vi "BRig_FPGA_v3,95__PortC.vi"() -> ()   [LabVIEW 2014]
uses:
  <vilib>/rvi/Emulation/niFpgaGetClockAttributes.vi
  <vilib>/rvi/Emulation/niFpgaSctlEmulationGetInTimedLoop.vi
  <vilib>/rvi/Emulation/niFpgaEmulationReportErrorSimple.vi
  <vilib>/rvi/eio/common/nirviEmuTemplateMethod_errors.vi
  <vilib>/rvi/Emulation/niFpgaCriticalErrorInLSC.vi
  <vilib>/eio/EIONode/EIONode.xnode
panel:
  out "AnaIn_1_0":i16
  out "AnaIn_1_1":i16
  out "AnaIn_1_2":i16
  out "AnaIn_1_3":i16
  out "AnaIn_1_4":i16
  out "AnaIn_0_4":i16
  out "AnaIn_0_3":i16
  out "AnaIn_0_2":i16
  out "AnaIn_0_1":i16
  out "AnaIn_0_0":i16
  in  "AI_newCycleFlag":bool
  in  "AnaOut1_Pair":u16
  in  "AnaOut0_Pair":u16
  out "fpga_solenoid_R":bool
  out "fpga_solenoid_L":bool
  out "fpga_laser2":bool
  out "fpga_laser1":bool
  in  "L2Led_ON":bool
  in  "L1Led_ON":bool
  in  "Rising(F)_or_Falling(T)":bool
  in  "Solenoid_trig_R":bool
  in  "Solenoid_trig_L":bool
  in  "Solenoid_nTotal_R":u32=100
  in  "Solenoid_nTotal_L":u32=100
  in  "L2Led_Baseline":bool
  in  "L1Led_Baseline":bool
  in  "CueLed_Baseline":bool
  in  "I_allReward":bool
  in  "AnaOut_1":i16
  in  "CueLed_Event":bool
  in  "CueLed_nValley":u32=100
  in  "CueLed_nPeak":u32=100
  in  "LC_Event_l2":bool
  in  "LC_Laser_l2":bool
  in  "LC_nShutter_l2":u32=100
  in  "LC_nValley_l2":u32=100
  in  "LC_nPeak_l2":u32=100
  in  "LR_wrong_nDelay_l2":u32
  in  "LR_reward_nDelay_l2":u32
  in  "LR_wrong_nTotal_l2":u32=100
  in  "LR_reward_nTotal_l2":u32=100
  in  "LR_wrong_laser_l2":bool
  in  "LR_wrong_Event_l2":bool
  in  "LR_reward_Laser_l2":bool
  in  "LR_reward_Event_l2":bool
  out "timeTrial_count":u32
  in  "timeTrial_trig":bool
  in  "k1__counter_per_ms":u16=100 min=100 max=40000 step=1
  in  "LC_nShutter_l1":u32=100
  in  "AnaOut_0":i16
  in  "LC_nValley_l1":u32=100
  in  "LC_nPeak_l1":u32=100
  in  "LC_Event_l1":bool
  in  "LR_wrong_nTotal_l1":u32=100
  in  "LR_wrong_nDelay_l1":u32
  in  "LR_reward_nTotal_l1":u32=100
  in  "LR_reward_nDelay_l1":u32
  in  "LR_reward_Event_l1":bool
  in  "LR_wrong_Event_l1":bool
  out "SelectWrong":bool
  out "SelectReward":bool
  in  "LR_wrong_Laser_l1":bool
  in  "LR_reward_Laser_l1":bool
  in  "Left(F)_or_Right(T)":bool
  in  "ignoreWrong":bool
  in  "SelectionState":bool
  in  "LC_Laser_l1":bool
  in  "FPGA_Stop":bool
  in  "audioTrigger_L":bool
  in  "audioTrigger_R":bool
  in  "audioFreq_L_kHz":u8=14 min=1 max=14 step=1
  in  "audioAmp_L":u16=1 min=1 max=32767 step=1
  in  "audioFreq_R_kHz":u8=14 min=1 max=14 step=1
  in  "audioAmp_R":u16=1 min=1 max=32767 step=1
  in  "A3_SL":bool
  in  "A1_SR":bool
  in  "Counts_Reset":bool
  out "A4_LickR":u32
  out "A2_LickL":u32
  in  "A6_Act":bool
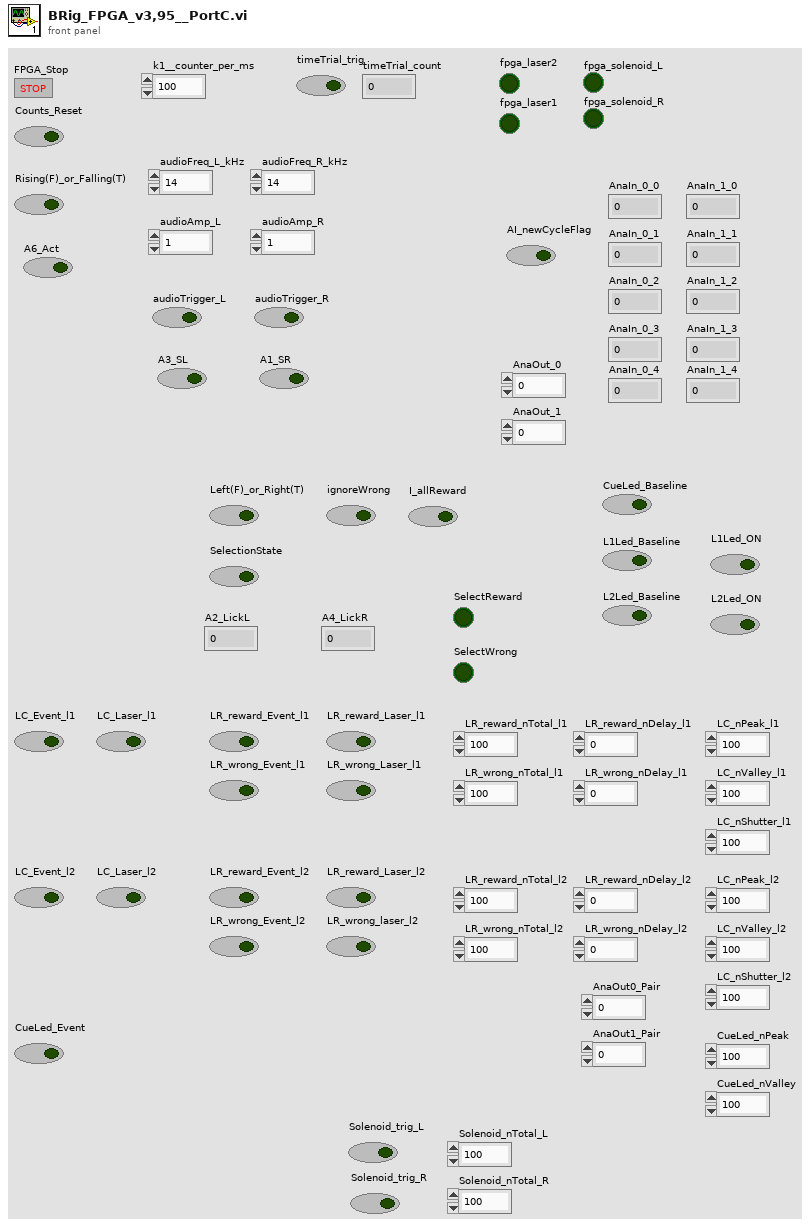
[diagram p1: front panel]
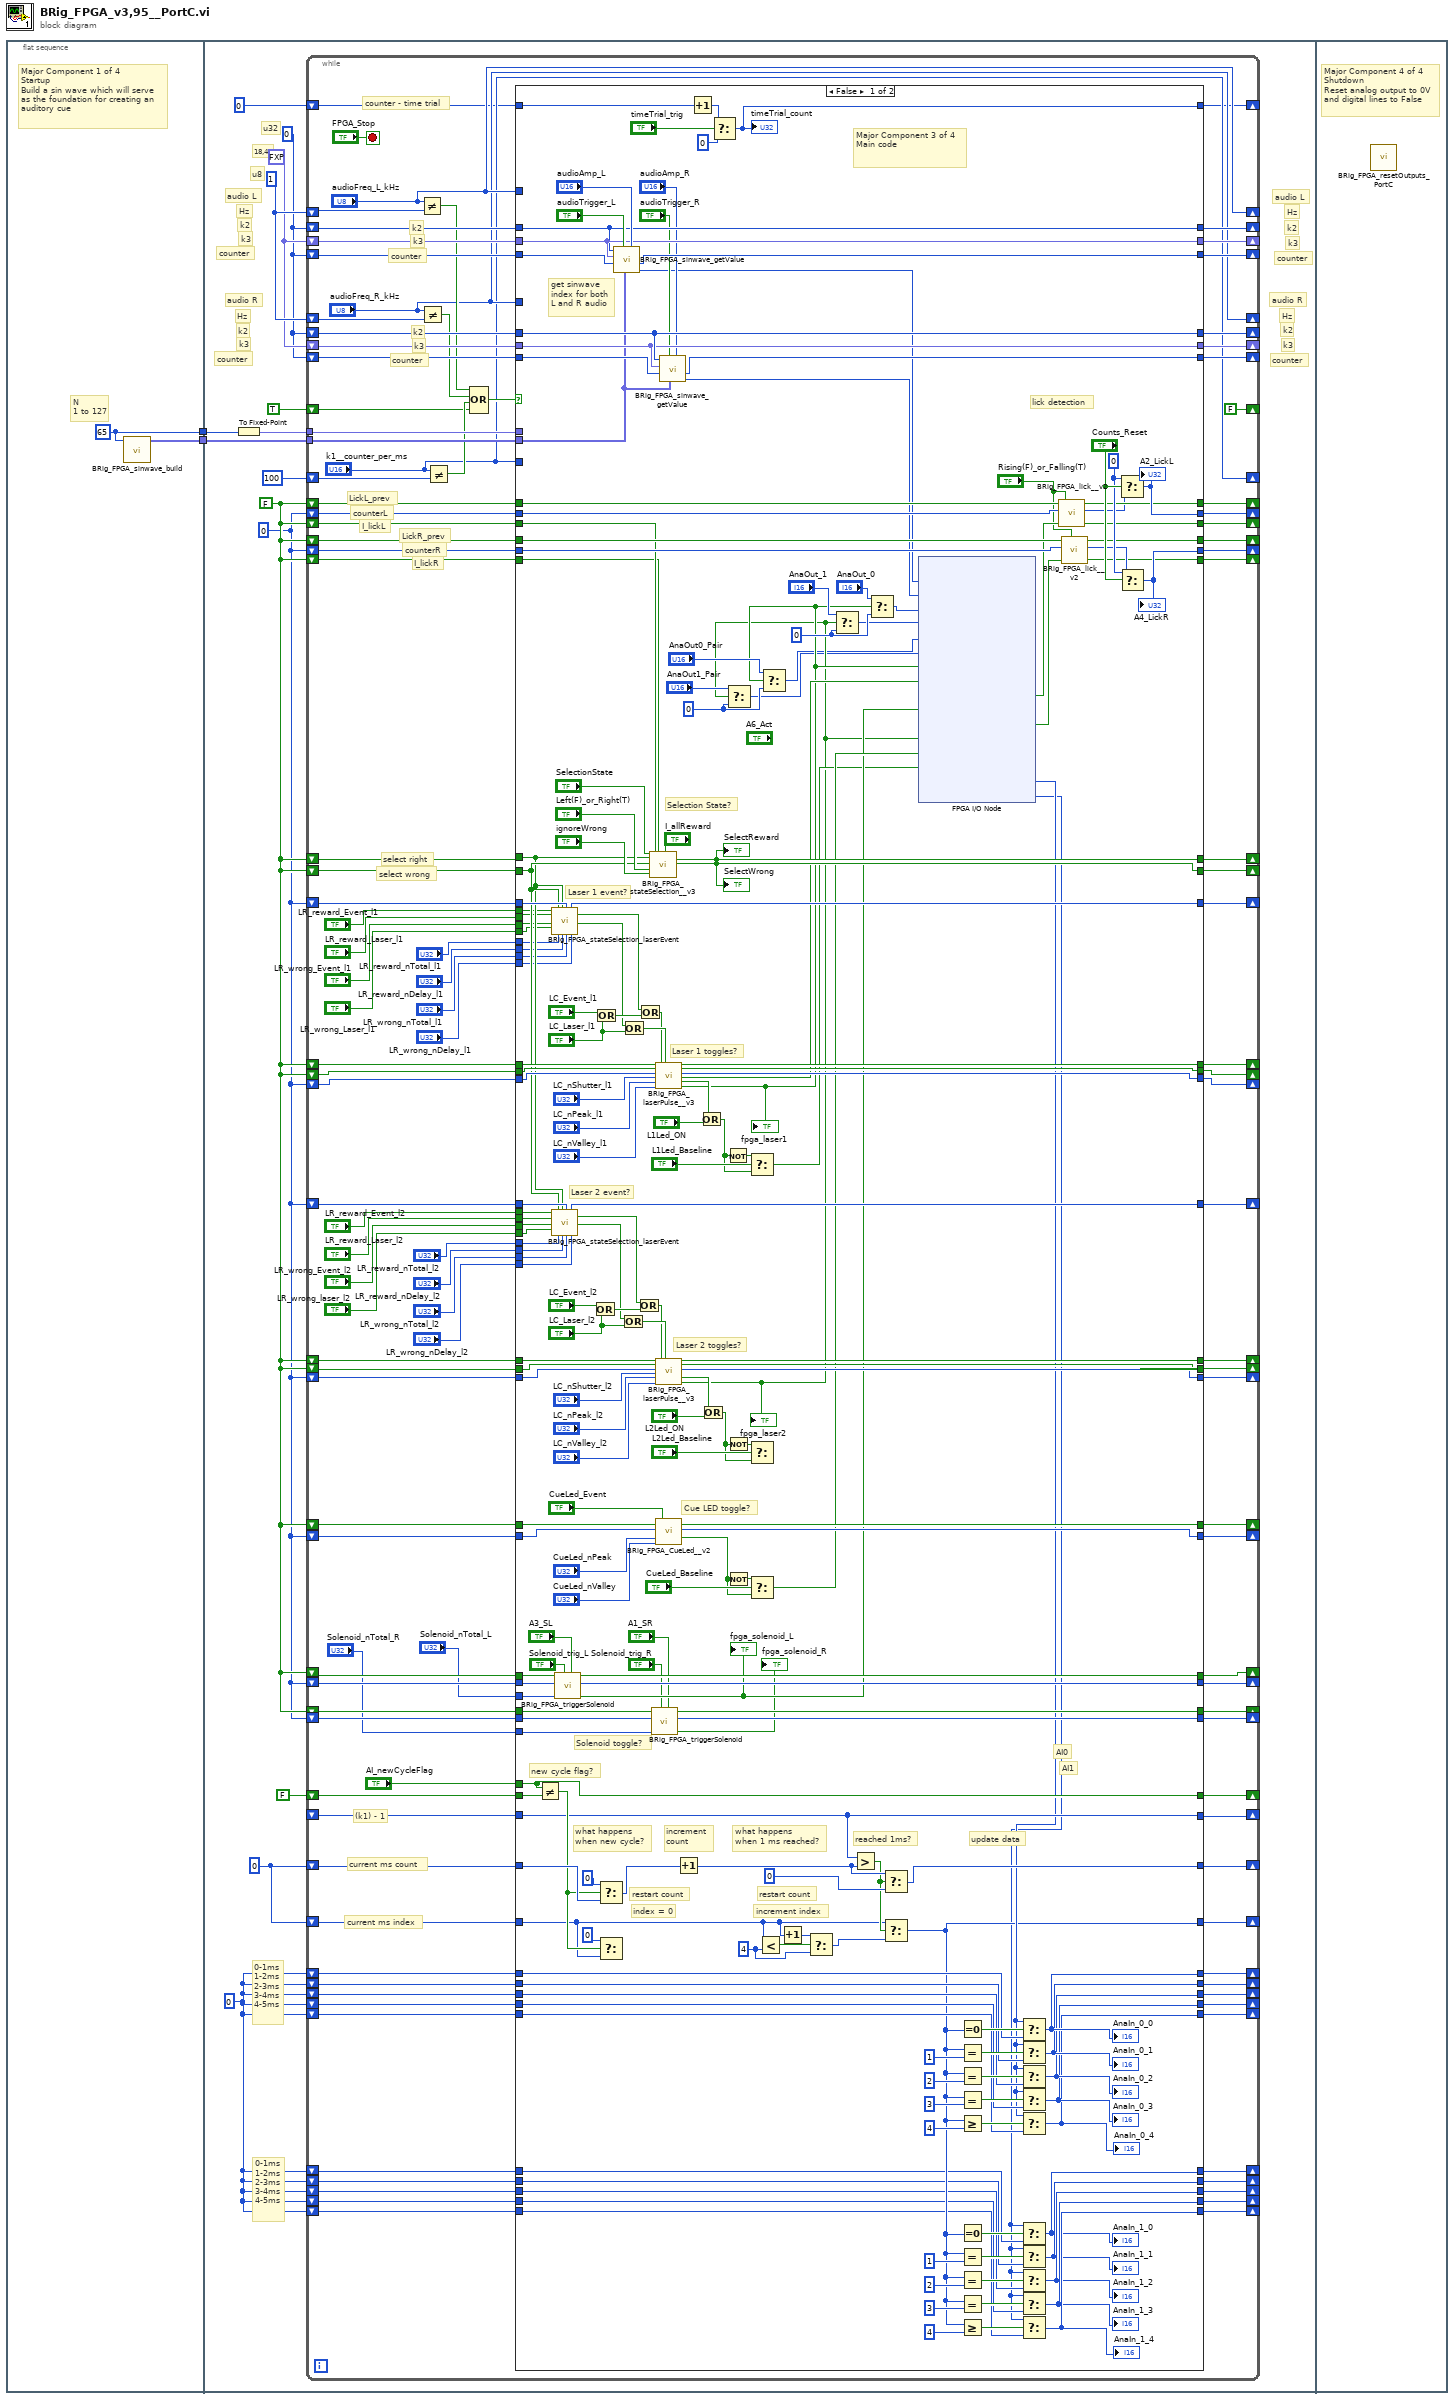
[diagram p0: block diagram]
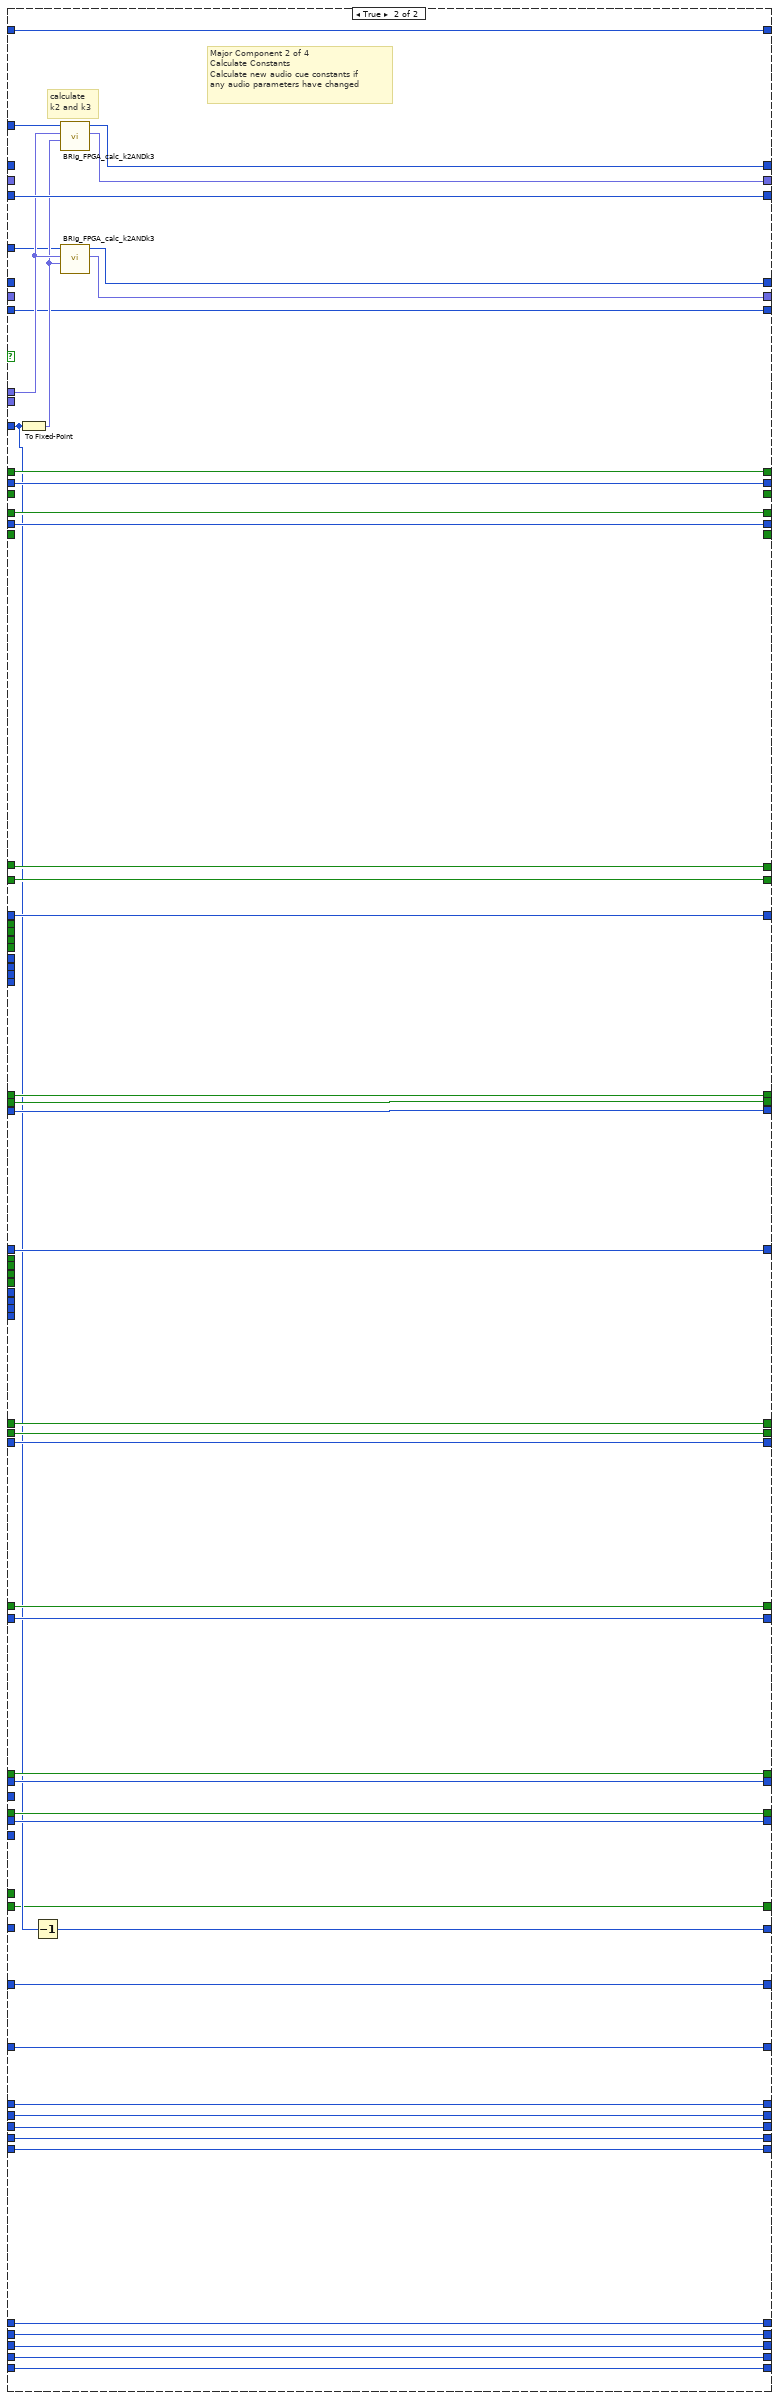
[diagram p2: hidden frame]
diagram:
  n1 = flat-sequence {
    tunnel: [w4] -> w2
    tunnel: [w3] -> w1
    tunnel: w2 -> [w18]
    tunnel: w1 -> [w17]
    frame #0 {
      w3 = 65 ("dimension size")
      # "Major Component 1 of 4\nStartup\nBuild a sin wave which will serve\nas the foundation for creating an\nauditory cue"
      # "N\n1 to 127"
      n2 = call "BRig_FPGA_sinwave_build.vi"("input_Npts"=w3) -> ("output_array_sin"=w4:fxp<+/-,16,2>[])  [unwired: 10 in]
    }
    frame #1 {
      w5 = i16 0
      w7 = u16 0
      w8 = u32 0
      w9 = FALSE
      w13 = u32 0
      w14 = fxp<+,18,4> 0.0
      w15 = u8 1
      # "0-1ms\n1-2ms\n2-3ms\n3-4ms\n4-5ms"
      # "0-1ms\n1-2ms\n2-3ms\n3-4ms\n4-5ms"
      # "counter"
      # "k3"
      # "k2"
      # "counter"
      # "k3"
      # "k2"
      # "counter"
      # "counter"
      # "u32"
      # "k3"
      # "k2"
      # "k3"
      # "18,4"
      # "u8"
      # "Hz"
      # "Hz"
      # "audio R"
      # "audio L"
      # "Hz"
      # "k2"
      # "Hz"
      # "audio R"
      # "audio L"
      n3 = To Fixed-Point(number=w17) -> (fixed-point=w16:fxp<+,7,7>)  [unwired: 1 in]
      n4 = while {
        shift-right: ["audioFreq_L_kHz"] -> _
        shift-left: w15 -> [w138]
        shift-right: [w132] -> _
        shift-left: w13 -> [w136]
        shift-right: ["audioFreq_R_kHz"] -> _
        shift-left: w15 -> [w128]
        tunnel: w18 -> [w135]
        tunnel: w16 -> [w134]
        shift-right: [w131] -> _
        shift-left: w14 -> [w133]
        shift-right: [w129] -> _
        shift-left: w13 -> [w130]
        shift-right: [w126] -> _
        shift-left: w13 -> [w127]
        shift-right: [w124] -> _
        shift-left: w14 -> [w125]
        shift-right: [w122] -> _
        shift-left: w13 -> [w123]
        shift-right: ["k1__counter_per_ms"] -> _
        shift-left: u16 100 ("y") -> [w121]
        shift-right: [FALSE] -> _
        shift-left: TRUE -> [w116]
        shift-right: [w109] -> _
        shift-left: w9 -> [w111]
        shift-right: [w108] -> _
        shift-left: w9 -> [w110]
        shift-right: [w106] -> _
        shift-left: w8 -> [w107]
        shift-right: [w104] -> _
        shift-left: w8 -> [w105]
        shift-right: [w101] -> _
        shift-left: w9 -> [w103]
        shift-right: [w100] -> _
        shift-left: w9 -> [w102]
        shift-right: [w98] -> _
        shift-left: w9 -> [w99]
        shift-right: [w96] -> _
        shift-left: w9 -> [w97]
        shift-right: [w94] -> _
        shift-left: u32 0 -> [w95]
        shift-right: [w92] -> _
        shift-left: w8 -> [w93]
        shift-right: [w91] -> _
        shift-left: w9 -> [w88]
        shift-right: [w90] -> _
        shift-left: w9 -> [w87]
        shift-right: [w89] -> _
        shift-left: w8 -> [w86]
        shift-right: [w84] -> _
        shift-left: w8 -> [w85]
        shift-right: [w83] -> _
        shift-left: w9 -> [w80]
        shift-right: [w82] -> _
        shift-left: w9 -> [w79]
        shift-right: [w81] -> _
        shift-left: w8 -> [w78]
        shift-right: [w77] -> _
        shift-left: w9 -> [w75]
        shift-right: [w76] -> _
        shift-left: w8 -> [w74]
        shift-right: [w56] -> _
        shift-left: w8 -> [w57]
        shift-right: [w53] -> _
        shift-left: w9 -> [w55]
        shift-right: [w50] -> _
        shift-left: w9 -> [w52]
        shift-right: [w49] -> _
        shift-left: w8 -> [w51]
        shift-right: [w47] -> _
        shift-left: _ -> [w46]
        shift-right: [w33] -> _
        shift-left: w7 -> [w45]
        shift-right: [w43] -> _
        shift-left: w5 -> [w44]
        shift-right: [w41] -> _
        shift-left: w5 -> [w42]
        shift-right: [w39] -> _
        shift-left: w5 -> [w40]
        shift-right: [w37] -> _
        shift-left: w5 -> [w38]
        shift-right: [w35] -> _
        shift-left: w5 -> [w36]
        shift-right: [w32] -> _
        shift-left: w7 -> [w34]
        shift-right: [w29] -> _
        shift-left: FALSE -> [w31]
        shift-right: [w27] -> _
        shift-left: w5 -> [w28]
        shift-right: [w25] -> _
        shift-left: w5 -> [w26]
        shift-right: [w23] -> _
        shift-left: w5 -> [w24]
        shift-right: [w22] -> _
        shift-left: w5 -> [w21]
        shift-right: [w20] -> _
        shift-left: w5 -> [w19]
        stop <- "FPGA_Stop" stop-if-true
        # "current ms index"
        # "current ms count"
        # "(k1) - 1"
        # "counter"
        # "k3"
        # "k2"
        # "counter"
        # "k3"
        # "k2"
        # "counter - time trial"
        # "I_lickR"
        # "counterR"
        # "LickR_prev"
        # "I_lickL"
        # "counterL"
        # "LickL_prev"
        # "select wrong"
        # "select right"
        n5 = Not Equal?(x="audioFreq_L_kHz", y=w138) -> (x != y?=w120:bool)
        n6 = Not Equal?(x="audioFreq_R_kHz", y=w128) -> (x != y?=w119:bool)
        n7 = Not Equal?(x="k1__counter_per_ms", y=w121) -> (x != y?=w117:bool)
        n8 = Compound Arithmetic op=OR(w120, w119, w117, w116) -> (w118:bool)
        n9 = case shown="False" w118 {
          tunnel: w136 -> [w331 _]
          tunnel: "audioFreq_L_kHz" -> [_ w392]
          tunnel: w135 -> [w324 _]
          tunnel: w134 -> [_ w388]
          tunnel: "k1__counter_per_ms" -> [_ w361]
          tunnel: w133 -> [w332 _]
          tunnel: [w331 w391] -> w132
          tunnel: [w332 w390] -> w131
          tunnel: w130 -> [w336 w389]
          tunnel: [w333 w389] -> w129
          tunnel: w127 -> [w328 _]
          tunnel: [w328 w384] -> w126
          tunnel: w125 -> [w327 _]
          tunnel: [w327 w385] -> w124
          tunnel: w123 -> [w330 w383]
          tunnel: "audioFreq_R_kHz" -> [_ w386]
          tunnel: [w329 w383] -> w122
          tunnel: w111 -> [w319 w382]
          tunnel: w110 -> [w318 w381]
          tunnel: [w323 w382] -> w109
          tunnel: [w316 w381] -> w108
          tunnel: w107 -> [w320 w380]
          tunnel: [w346 w380] -> w106
          tunnel: w105 -> [w317 w379]
          tunnel: [w343 w379] -> w104
          tunnel: w103 -> [w272 w378]
          tunnel: w102 -> [w273 w377]
          tunnel: [w292 w378] -> w101
          tunnel: [w339 w377] -> w100
          tunnel: [w309 w374] -> w91
          tunnel: [w310 w373] -> w90
          tunnel: [w311 w372] -> w89
          tunnel: w99 -> [w313 _]
          tunnel: [w322 _] -> w98
          tunnel: w97 -> [w312 _]
          tunnel: [w314 _] -> w96
          tunnel: w95 -> [w301 w376]
          tunnel: [w298 w376] -> w94
          tunnel: w93 -> [w291 w375]
          tunnel: [w290 w375] -> w92
          tunnel: w88 -> [w289 w374]
          tunnel: w87 -> [w288 w373]
          tunnel: w86 -> [w287 w372]
          tunnel: w85 -> [w275 w371]
          tunnel: [w274 w371] -> w84
          tunnel: [w270 w370] -> w83
          tunnel: [w269 w369] -> w82
          tunnel: [w268 w368] -> w81
          tunnel: w80 -> [w267 w370]
          tunnel: w79 -> [w266 w369]
          tunnel: w78 -> [w265 w368]
          tunnel: [w262 w367] -> w77
          tunnel: [w261 w366] -> w76
          tunnel: w75 -> [w260 w367]
          tunnel: w74 -> [w259 w366]
          tunnel: "LR_reward_Event_l1" -> [w244 _]
          tunnel: "LR_reward_Laser_l1" -> [w243 _]
          tunnel: "LR_wrong_Event_l1" -> [w242 _]
          tunnel: "LR_wrong_Laser_l1" -> [w241 _]
          tunnel: "LR_reward_nTotal_l1" -> [w240 _]
          tunnel: "LR_reward_nDelay_l1" -> [w239 _]
          tunnel: "LR_wrong_nTotal_l1" -> [w238 _]
          tunnel: "LR_wrong_nDelay_l1" -> [w237 _]
          tunnel: "LR_reward_Event_l2" -> [w236 _]
          tunnel: "LR_reward_Laser_l2" -> [w235 _]
          tunnel: "LR_wrong_Event_l2" -> [w234 _]
          tunnel: "LR_wrong_laser_l2" -> [w233 _]
          tunnel: "LR_reward_nTotal_l2" -> [w232 _]
          tunnel: "LR_reward_nDelay_l2" -> [w231 _]
          tunnel: "LR_wrong_nTotal_l2" -> [w230 _]
          tunnel: "LR_wrong_nDelay_l2" -> [w229 _]
          tunnel: w57 -> [w228 w365]
          tunnel: [w223 w365] -> w56
          tunnel: w55 -> [w227 w364]
          tunnel: "Solenoid_nTotal_L" -> [w226 _]
          tunnel: [w222 w364] -> w53
          tunnel: w52 -> [w218 w363]
          tunnel: w51 -> [w217 w362]
          tunnel: [w216 w363] -> w50
          tunnel: [w215 w362] -> w49
          tunnel: "Solenoid_nTotal_R" -> [w214 _]
          tunnel: [w187 w360] -> w47
          tunnel: w46 -> [w187 _]
          tunnel: w45 -> [w191 w359]
          tunnel: [w180 w359] -> w33
          tunnel: w44 -> [w170 w358]
          tunnel: [w165 w358] -> w43
          tunnel: w42 -> [w168 w357]
          tunnel: [w164 w357] -> w41
          tunnel: w40 -> [w169 w356]
          tunnel: [w163 w356] -> w39
          tunnel: w38 -> [w167 w355]
          tunnel: [w162 w355] -> w37
          tunnel: w36 -> [w166 w354]
          tunnel: [w161 w354] -> w35
          tunnel: w34 -> [w183 w353]
          tunnel: [w150 w353] -> w32
          tunnel: w31 -> [w196 w352]
          tunnel: "AI_newCycleFlag" -> [w195 _]
          tunnel: [w195 w352] -> w29
          tunnel: w28 -> [w145 w351]
          tunnel: [w140 w351] -> w27
          tunnel: w26 -> [w146 w350]
          tunnel: [w141 w350] -> w25
          tunnel: w24 -> [w147 w349]
          tunnel: [w142 w349] -> w23
          tunnel: [w143 w348] -> w22
          tunnel: w21 -> [w148 w348]
          tunnel: [w144 w347] -> w20
          tunnel: w19 -> [w149 w347]
          frame False {
            w181 = u16 4 ("y")
            w202 = u16 0 ("f")
            w256 = i16 0 ("f")
            w344 = u32 0 ("t")
            # "increment index"
            # "restart count"
            # "index = 0"
            # "restart count"
            # "AI1"
            # "AI0"
            # "update data"
            # "reached 1ms?"
            # "increment\ncount"
            # "what happens\nwhen new cycle?"
            # "what happens\nwhen 1 ms reached?"
            # "new cycle flag?"
            # "Solenoid toggle?"
            # "Cue LED toggle?"
            # "Laser 2 toggles?"
            # "Laser 2 event?"
            # "Laser 1 toggles?"
            # "Selection State?"
            # "Laser 1 event?"
            # "Major Component 3 of 4\nMain code"
            # "get sinwave\nindex for both\nL and R audio"
            # "lick detection"
            n10 = Not Equal?(x=w195, y=w196) -> (x != y?=w189:bool)
            n11 = call "BRig_FPGA_stateSelection_laserEvent.vi"("I_LR_reward"=w244, "I_LR_reward_laser"=w243, "I_LR_wrong"=w242, "I_LR_wrong_laser"=w241, "I_selectWrong"=w273, "laser_reward_nTotal"=w240, "I_selectReward"=w272, "laser_reward_nDelay"=w239, "counter"=w291, "laser_wrong_nTotal"=w238, "laser_wrong_nDelay"=w237) -> ("output_counter"=w290:u32, "output_I_laserEvent"=w286:bool, "output_I_laserOn"=w285:bool)  [unwired: 6 in]
            n12 = call "BRig_FPGA_stateSelection_laserEvent.vi"("I_LR_reward"=w236, "I_LR_reward_laser"=w235, "I_LR_wrong"=w234, "I_LR_wrong_laser"=w233, "I_selectWrong"=w273, "laser_reward_nTotal"=w232, "I_selectReward"=w272, "laser_reward_nDelay"=w231, "counter"=w275, "laser_wrong_nTotal"=w230, "laser_wrong_nDelay"=w229) -> ("output_counter"=w274:u32, "output_I_laserEvent"=w271:bool, "output_I_laserOn"=w276:bool)  [unwired: 6 in]
            n13 = call "BRig_FPGA_triggerSolenoid.vi"("input_Solenoid_MTrig"="A3_SL", "input_Solenoid_trig"="Solenoid_trig_L", "input_threshold"=w226, "input_counter"=w228, "input_trig"=w227) -> ("output_Solenoid_OnOff"=w221:bool, "output_counter"=w223:u32, "output_trig"=w222:bool)  [unwired: 4 in]
            "fpga_solenoid_L" <- w221
            n14 = Or(x="LC_Event_l2", y="LC_Laser_l2") -> (x .or. y?=w280:bool)
            n15 = Or(x="LC_Event_l1", y="LC_Laser_l1") -> (x .or. y?=w305:bool)
            n16 = Select(t=u16 0, s=w189, f=w191) -> (s? t:f=w188:u16)
            n17 = Select(t=u16 0 ("f"), s=w189, f=w183) -> ()  [unwired: 1 out]
            n18 = call "BRig_FPGA_sinwave_getValue.vi"("audioAmp"="audioAmp_L", "sinwave"=w324, "audioTrigger"="audioTrigger_L", "counter"=w336, "k3"=w332, "k2"=w331) -> ("output_audioValue"=w296:i16, "output_counter"=w333:u32)  [unwired: 4 in]
            n19 = Or(x=w276, y="LC_Laser_l2") -> (x .or. y?=w278:bool)
            n20 = Or(x=w285, y="LC_Laser_l1") -> (x .or. y?=w303:bool)
            n21 = Or(x=w271, y=w280) -> (x .or. y?=w277:bool)
            n22 = Or(x=w286, y=w305) -> (x .or. y?=w302:bool)
            n23 = call "BRig_FPGA_stateSelection__v3.vi"("I_selectionState"="SelectionState", "I_selectRight"=w272, "I_selectWrong"=w273, "I_Left(F)_or_Right(T)"="Left(F)_or_Right(T)", "I_ignoreWrong"="ignoreWrong", "I_lickL"=w313, "I_lickR"=w312, "I_allReward"="I_allReward") -> ("output__I_selectRight"=w292:bool, "output__I_selectWrong"=w339:bool)  [unwired: 18 in]
            "SelectWrong" <- w339
            "SelectReward" <- w292
            n24 = call "BRig_FPGA_triggerSolenoid.vi"("input_Solenoid_MTrig"="A1_SR", "input_Solenoid_trig"="Solenoid_trig_R", "input_threshold"=w214, "input_counter"=w217, "input_trig"=w218) -> ("output_Solenoid_OnOff"=→"fpga_solenoid_R":bool, "output_counter"=w215:u32, "output_trig"=w216:bool)  [unwired: 4 in]
            n25 = call "BRig_FPGA_laserPulse__v3.vi"("I_shutter"=w289, "I_peak"=w288, "count"=w287, "laser_Nshutter"="LC_nShutter_l1", "laser_Npeak"="LC_nPeak_l1", "laser_Nvalley"="LC_nValley_l1", "I_laserEvent"=w302, "I_laser"=w303) -> ("output_I_shutter"=w309:bool, "output_I_peak"=w310:bool, "output_count"=w311:u32, "output_shutter"=w205:bool, "output_led"=w210:bool, "output_laser"=w200:bool)  [unwired: 6 in]
            "fpga_laser1" <- w200
            n26 = call "BRig_FPGA_laserPulse__v3.vi"("I_shutter"=w267, "I_peak"=w266, "count"=w265, "laser_Nshutter"="LC_nShutter_l2", "laser_Npeak"="LC_nPeak_l2", "laser_Nvalley"="LC_nValley_l2", "I_laserEvent"=w277, "I_laser"=w278) -> ("output_I_shutter"=w270:bool, "output_I_peak"=w269:bool, "output_count"=w268:u32, "output_led"=w207:bool, "output_laser"=w199:bool)  [unwired: 6 in, 1 out]
            "fpga_laser2" <- w199
            n27 = call "BRig_FPGA_CueLed__v2.vi"("I_peak"=w260, "count"=w259, "laser_Npeak"="CueLed_nPeak", "laser_Nvalley"="CueLed_nValley", "I_CueLed_Event"="CueLed_Event") -> ("output_I_peak"=w262:bool, "output_count"=w261:u32, "output_led"=w249:bool)  [unwired: 12 in]
            n28 = call "BRig_FPGA_sinwave_getValue.vi"("audioAmp"="audioAmp_R", "sinwave"=w324, "audioTrigger"="audioTrigger_R", "counter"=w330, "k3"=w327, "k2"=w328) -> ("output_audioValue"=w295:i16, "output_counter"=w329:u32)  [unwired: 4 in]
            n29 = Increment(x=w188) -> (x+1=w186:u16)
            n30 = Increment(x=w301) -> (x+1=w300:u32)
            n31 = Or(x=w210, y="L1Led_ON") -> (x .or. y?=w209:bool)
            n32 = Or(x=w207, y="L2Led_ON") -> (x .or. y?=w206:bool)
            n33 = Select(t=w300, s="timeTrial_trig", f=u32 0) -> (s? t:f=w298:u32)
            "timeTrial_count" <- w298
            n34 = Not(x=w209) -> (.not. x?=w248:bool)
            n35 = Select(t="AnaOut1_Pair", s=w199, f=w202) -> (s? t:f=w198:u16)
            n36 = Not(x=w206) -> (.not. x?=w246:bool)
            n37 = Not(x=w249) -> (.not. x?=w251:bool)
            n38 = Select(t=w248, s="L1Led_Baseline", f=w209) -> (s? t:f=w212:bool)
            n39 = Select(t=w246, s="L2Led_Baseline", f=w206) -> ()  [unwired: 1 out]
            n40 = Select(t=w251, s="CueLed_Baseline", f=w249) -> (s? t:f=w252:bool)
            n41 = Less?(x=w183, y=w181) -> (x < y?=w194:bool)
            n42 = Select(t="AnaOut0_Pair", s=w200, f=w202) -> (s? t:f=w197:u16)
            n43 = Increment(x=w183) -> (x+1=w193:u16)
            n44 = Select(t=w193, s=w194, f=w181) -> (s? t:f=w182:u16)
            n45 = Select(t="AnaOut_1", s=w199, f=w256) -> (s? t:f=w254:i16)
            n46 = Greater?(x=w187, y=w186) -> (0:w184:bool)
            n47 = Select(t="AnaOut_0", s=w200, f=w256) -> (s? t:f=w257:i16)
            n48 = Select(t=w186, s=w184, f=u16 0) -> (s? t:f=w180:u16)
            n49 = Select(t=w183, s=w184, f=w182) -> (s? t:f=w150:u16)
            n50 = xnode "FPGA I/O Node"("AudioOut/Left"=w296, "AudioOut/Right"=w295, "ConnectorC/AO0"=w257, "ConnectorC/AO1"=w254, "ConnectorB/AO0"=w197, "ConnectorB/AO1"=w198, "ConnectorC/DIO0"=w200, "ConnectorC/DIO1"=w205, "ConnectorC/DIO3"=w221, "ConnectorC/DIO5"=w199, "ConnectorC/DIO6"=w252, "ConnectorC/DIO7"=w212) -> ("ConnectorC/DIO2"=w294:bool, "ConnectorC/DIO4"=w293:bool, "ConnectorC/AI0"=w151:i16, "ConnectorC/AI1"=w139:i16)  [unwired: 16 in, 16 out]
            n51 = Equal To 0?(x=w150) -> (x = 0?=w179:bool)
            n52 = Equal?(x=w150, y=u16 1) -> (x = y?=w174:bool)
            n53 = Equal?(x=w150, y=u16 2) -> (x = y?=w173:bool)
            n54 = Equal?(x=w150, y=u16 3) -> (x = y?=w172:bool)
            n55 = Greater Or Equal?(x=w150, y=u16 4) -> (x >= y?=w171:bool)
            n56 = Equal To 0?(x=w150) -> (x = 0?=w152:bool)
            n57 = Equal?(x=w150, y=u16 1) -> (x = y?=w157:bool)
            n58 = Equal?(x=w150, y=u16 2) -> (x = y?=w158:bool)
            n59 = Equal?(x=w150, y=u16 3) -> (x = y?=w159:bool)
            n60 = Greater Or Equal?(x=w150, y=u16 4) -> (x >= y?=w160:bool)
            n61 = Select(t=w151, s=w179, f=w170) -> (s? t:f=w165:i16)
            "AnaIn_0_0" <- w165
            n62 = Select(t=w151, s=w174, f=w168) -> (s? t:f=w164:i16)
            "AnaIn_0_1" <- w164
            n63 = Select(t=w151, s=w173, f=w169) -> (s? t:f=w163:i16)
            "AnaIn_0_2" <- w163
            n64 = Select(t=w151, s=w172, f=w167) -> (s? t:f=w162:i16)
            "AnaIn_0_3" <- w162
            n65 = Select(t=w151, s=w171, f=w166) -> (s? t:f=w161:i16)
            "AnaIn_0_4" <- w161
            n66 = Select(t=w139, s=w152, f=w145) -> (s? t:f=w140:i16)
            "AnaIn_1_0" <- w140
            n67 = Select(t=w139, s=w157, f=w146) -> (s? t:f=w141:i16)
            "AnaIn_1_1" <- w141
            n68 = Select(t=w139, s=w158, f=w147) -> (s? t:f=w142:i16)
            "AnaIn_1_2" <- w142
            n69 = Select(t=w139, s=w159, f=w148) -> (s? t:f=w143:i16)
            "AnaIn_1_3" <- w143
            n70 = Select(t=w139, s=w160, f=w149) -> (s? t:f=w144:i16)
            "AnaIn_1_4" <- w144
            n71 = call "BRig_FPGA_lick__v2.vi"("Rising(F)_or_Falling(T)"="Rising(F)_or_Falling(T)", "I_stateDetector_new"=w294, "counter"=w320, "I_stateDetector_prev"=w319) -> ("output_I_lick"=w322:bool, "output_counter"=w321:u32, "output_I_stateDetector_prev"=w323:bool)  [unwired: 5 in]
            n72 = call "BRig_FPGA_lick__v2.vi"("Rising(F)_or_Falling(T)"="Rising(F)_or_Falling(T)", "I_stateDetector_new"=w293, "counter"=w317, "I_stateDetector_prev"=w318) -> ("output_I_lick"=w314:bool, "output_counter"=w315:u32, "output_I_stateDetector_prev"=w316:bool)  [unwired: 5 in]
            n73 = Select(t=w344, s="Counts_Reset", f=w321) -> (s? t:f=w346:u32)
            "A2_LickL" <- w346
            n74 = Select(t=w344, s="Counts_Reset", f=w315) -> (s? t:f=w343:u32)
            "A4_LickR" <- w343
          }
          frame True {
            # "Major Component 2 of 4\nCalculate Constants\nCalculate new audio cue constants if\nany audio parameters have changed"
            # "calculate\nk2 and k3"
            n75 = To Fixed-Point(number=w361) -> (fixed-point=w387:fxp<+,16,16>)  [unwired: 1 in]
            n76 = Decrement(x=w361) -> (x-1=w360:u16)
            n77 = call "BRig_FPGA_calc_k2ANDk3.vi"("input_k1[count/ms]"=w387, "input_Npts"=w388, "input_freq[kHz]"=w392) -> ("output_k3"=w390:fxp<+,18,4>, "output_k2"=w391:u32)  [unwired: 7 in]
            n78 = call "BRig_FPGA_calc_k2ANDk3.vi"("input_k1[count/ms]"=w387, "input_Npts"=w388, "input_freq[kHz]"=w386) -> ("output_k3"=w385:fxp<+,18,4>, "output_k2"=w384:u32)  [unwired: 7 in]
          }
        }
      }
    }
    frame #2 {
      # "Major Component 4 of 4\nShutdown\nReset analog output to 0V\nand digital lines to False"
      n79 = call "BRig_FPGA_resetOutputs_PortC.vi"() -> ()  [unwired: 12 in]
    }
  }
